vi "Helper SubVI - Get Signal-to-noise Ratio (SNR).vi"(10 "noisy signal":dbl[](array[numeric]), 11 "signal":dbl[](array[numeric])) -> (3 "SNR (dB)":dbl)   [LabVIEW 2023]
doc: "Computes the signal-to-noise ratio (SNR) of the reconstructed signal."
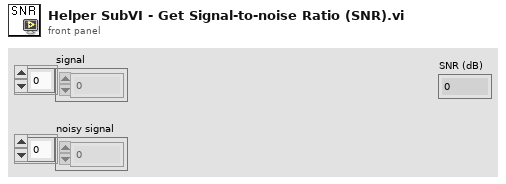
[diagram p1: front panel]
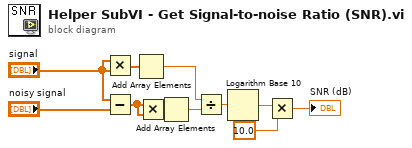
[diagram p0: block diagram]
diagram:
  n1 = Multiply(x="signal", y="signal") -> (x*y=w4:dbl[])
  n2 = Subtract(x="signal", y="noisy signal") -> (x-y=w3:dbl[])
  n3 = Add Array Elements(numeric array=w4) -> (sum=w10:dbl)
  n4 = Multiply(x=w3, y=w3) -> (x*y=w5:dbl[])
  n5 = Add Array Elements(numeric array=w5) -> (sum=w11:dbl)
  n6 = Divide(x=w10, y=w11) -> (x/y=w6:dbl)
  n7 = Logarithm Base 10(1:w6) -> (0:w7:dbl)
  n8 = Multiply(x=w7, y=10.0) -> (x*y=→"SNR (dB)":dbl)
